vi "Day09-01_비전과 모션.vi"() -> ()   [LabVIEW 2021]
uses:
  <vilib>/userDefined/High Color/IMAQdx.ctl
  <vilib>/vision/driver/NI_Vision_Acquisition_Software.lvlib
  <vilib>/vision/NI_Vision_Development_Module.lvlib
panel:
  out "Image 3":T1(plugin-control)
  out "색상":enum16{"모름", "빨강", "초록", "노랑", "파랑", "보라", "하늘"}(ring)
  out "히스토그램":u8[][](graph)
  in  "수집 3":bool
  in  "정지 3":bool
  out "Image 2":T1(plugin-control)
  in  "정지 2":bool
  out "웨이브폼 그래프":u32[][](graph)
  in  "수집":bool
  in  "정지":bool
  out "Image":T1(plugin-control)
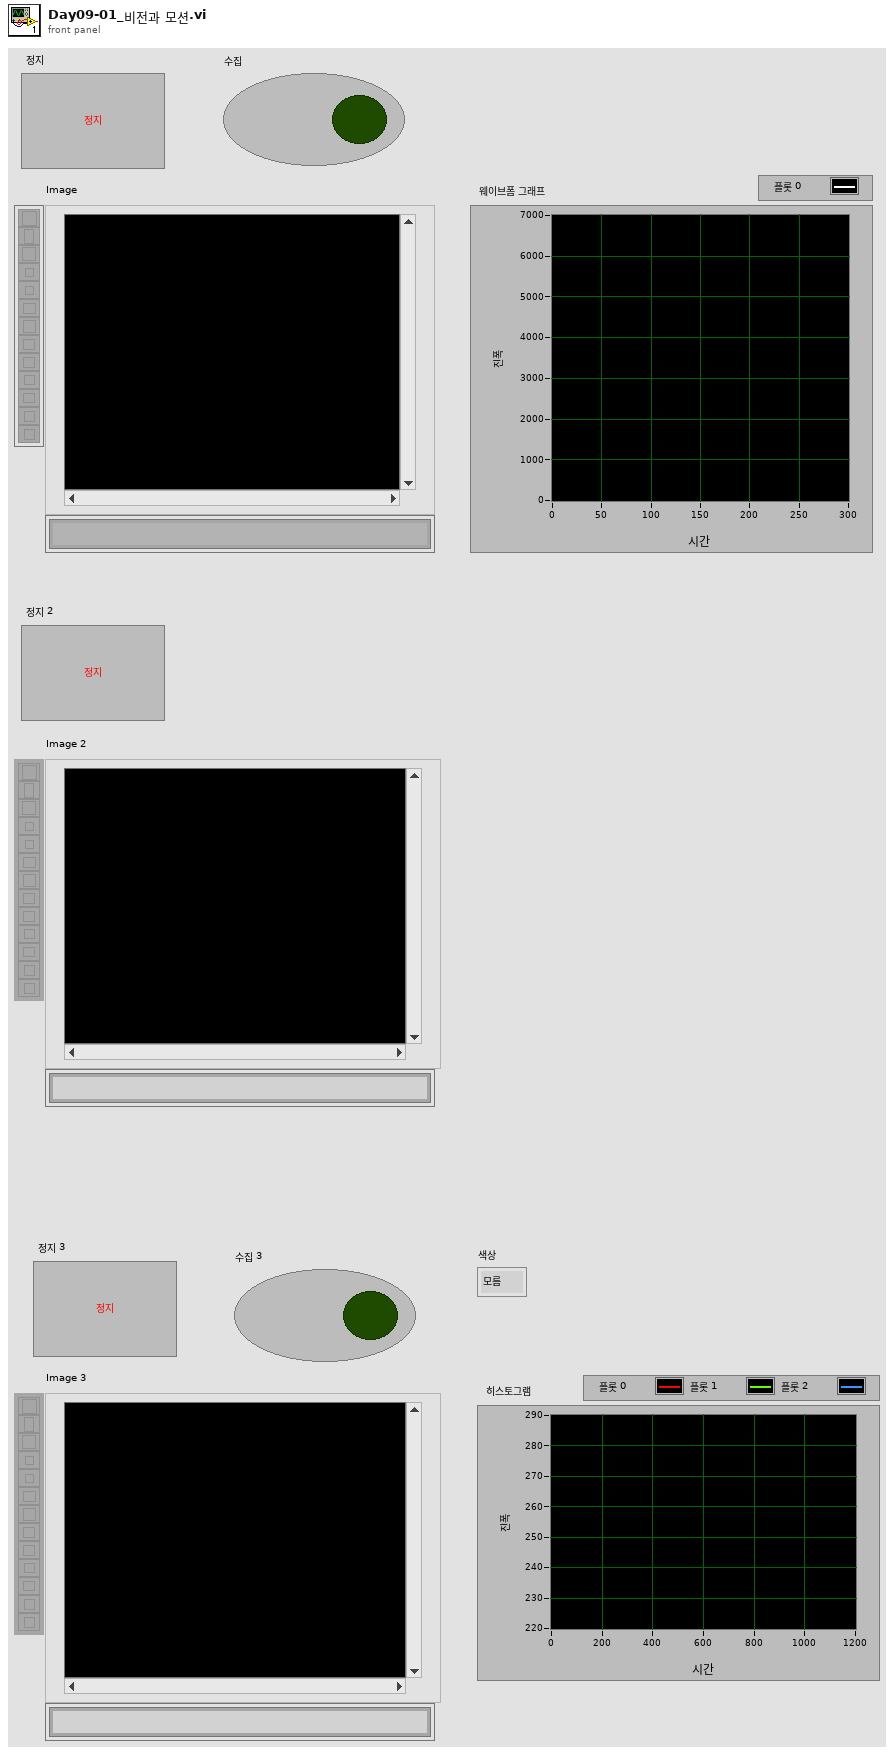
[diagram p1: front panel]
types:
  T1 = typedef "IMAQ Image.ctl" = refnum<image>
  T2 = typedef "IMAQdx.ctl" = refnum<k21>
  T3 = typedef "ROI Descriptor" = cluster{"Global Rectangle":i32[], "Contours":cluster{"ID":enum32{"External", "Internal"}, "Type":u32, "Coordinates":i32[]}[]}
  T4 = cluster{"histogram":u32[], "Minimal Value":sgl, "Maximal Value":sgl, "Starting Value":sgl, "Interval Width":sgl, "Mean Value":sgl, "Standard  Variation":sgl, "Area (pixels)":i32}
  T5 = enum16{"모름", "빨강", "초록", "노랑", "파랑", "보라", "하늘", "흰색"}[]
  T6 = enum16{"모름", "빨강", "초록", "노랑", "파랑", "보라", "하늘", "흰색"}
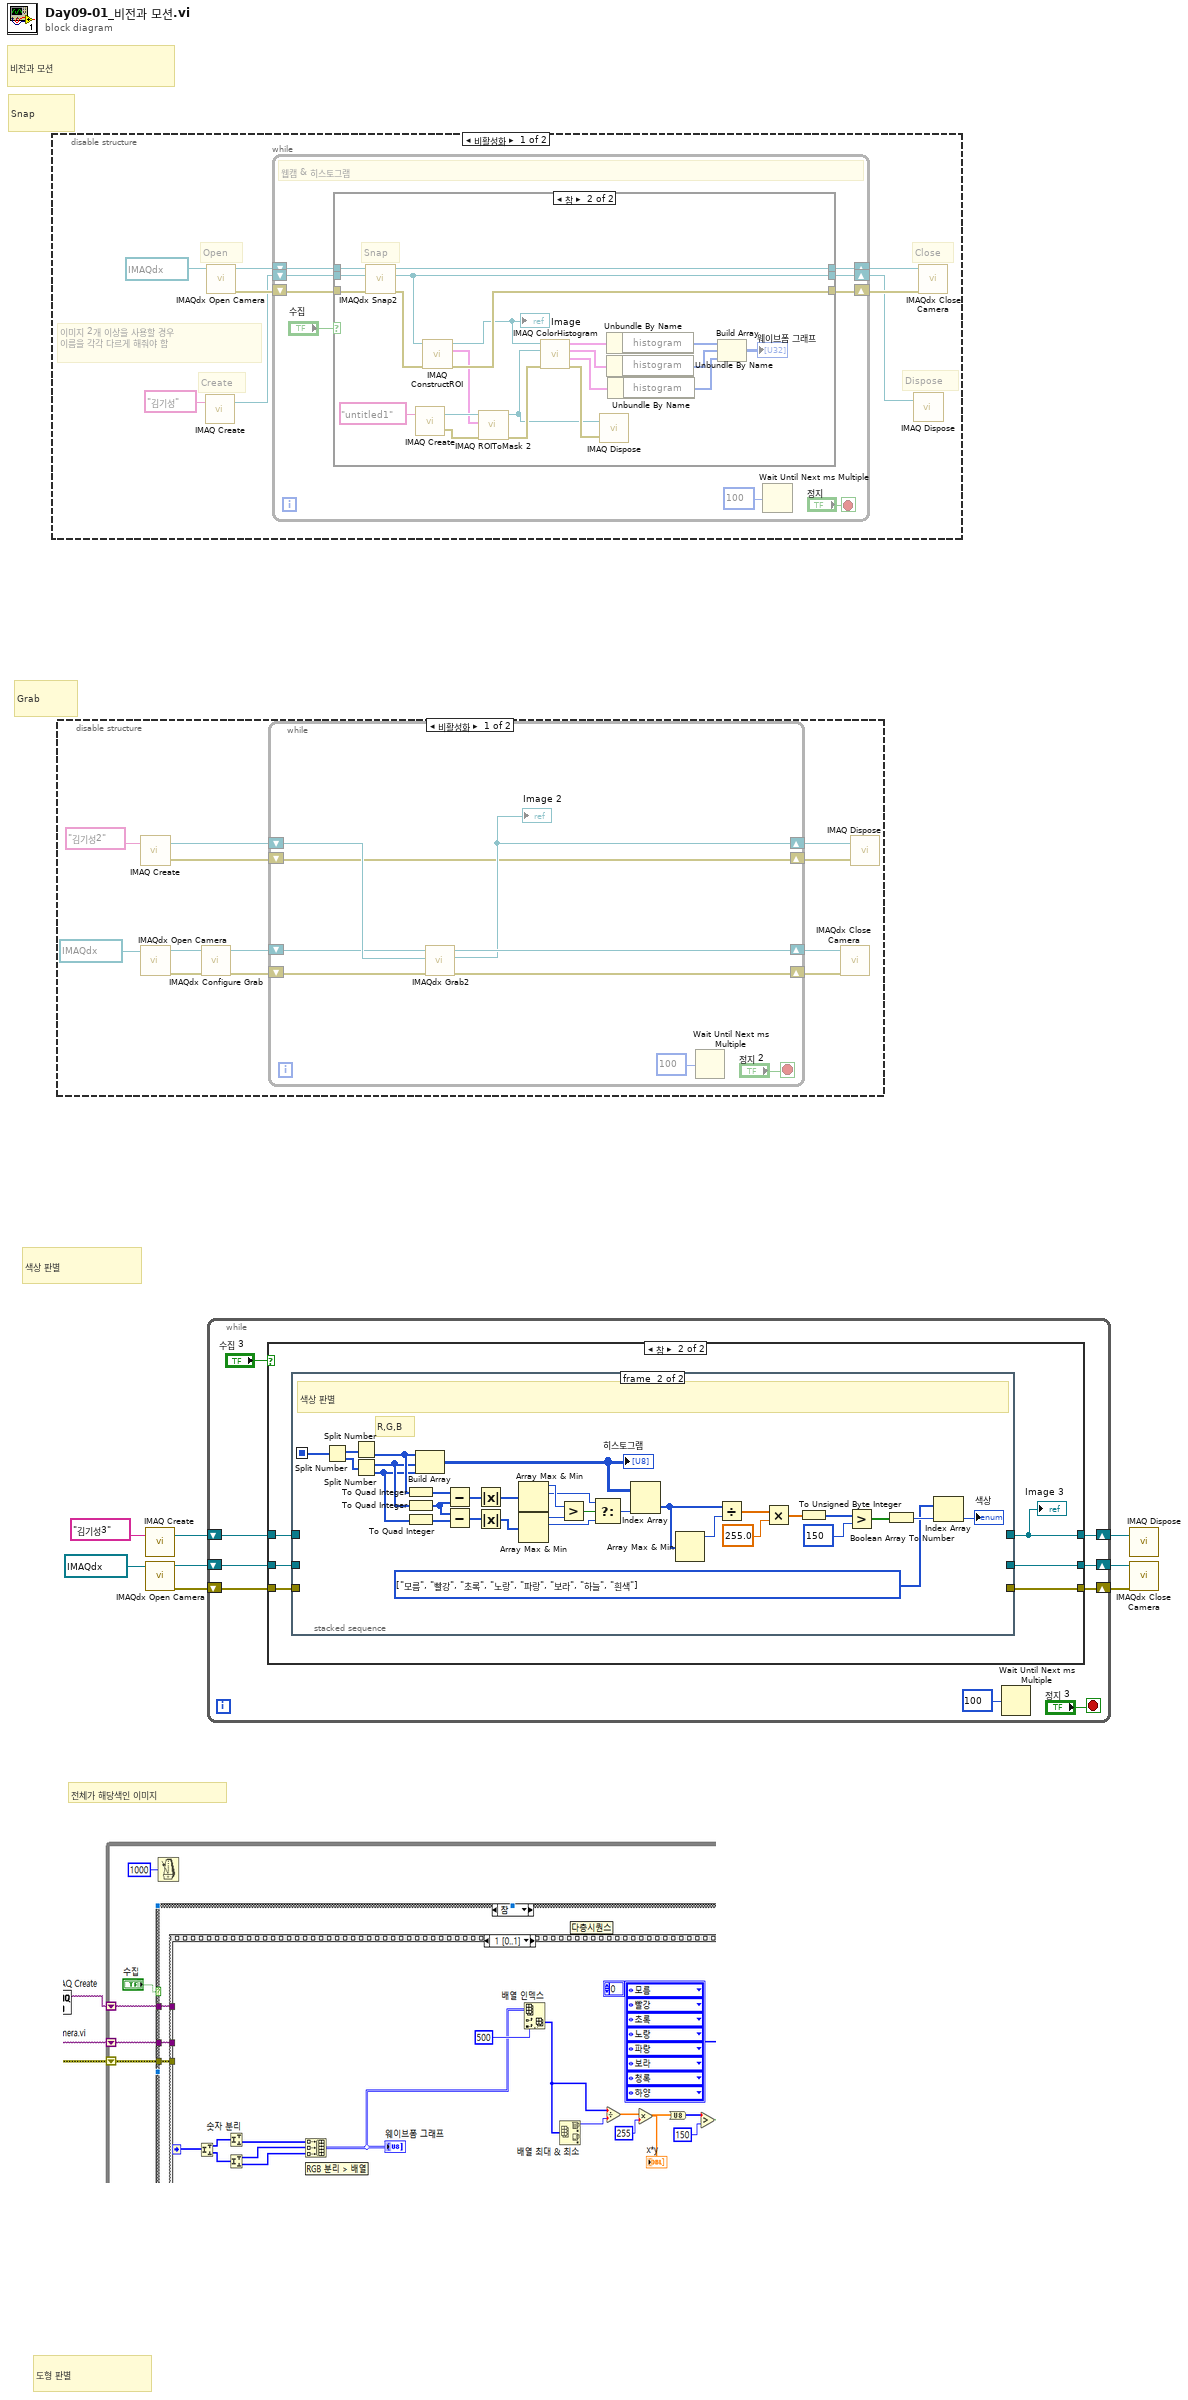
[diagram p0: block diagram]
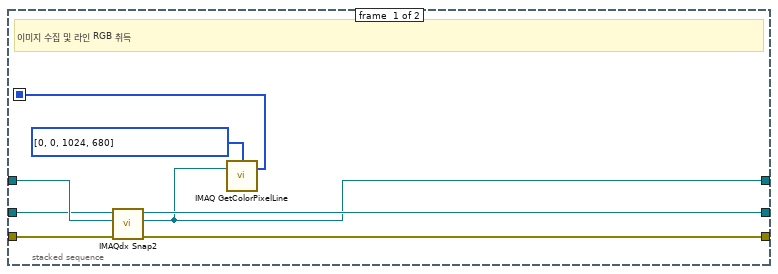
[diagram p4: hidden frame]
diagram:
  # "전체가 해당색인 이미지"
  # "도형 판별"
  # "색상 판별"
  # "Snap"
  # "Grab"
  # "비전과 모션"
  n1 = disable-structure shown="비활성화" {
    frame Disabled {
      # "Dispose"
      # "이미지 2개 이상을 사용할 경우\n이름을 각각 다르게 해줘야 함"
      # "Create"
      # "Close"
      # "Open"
      n2 = call "IMAQ Create"("Image Name"="김기성") -> ("New Image"=w10:T1)  [unwired: 4 in, 1 out]
      n3 = call <vilib>:"IMAQdx Open Camera.vi"("Session In"=T2 "cam1") -> ("error out"=w15:errorcluster, "Session Out"=w16:T2)  [unwired: 9 in]
      n4 = while {
        shift-right: [w23] -> w14
        shift-left: w16 -> [w25]
        shift-right: [w22] -> w13
        shift-left: w15 -> [w24]
        shift-right: [w18] -> w9
        shift-left: w10 -> [w21]
        stop <- "정지" stop-if-true
        # "웹캠 & 히스토그램"
        n5 = case shown="참" "수집" {
          tunnel: w25 -> [w28 w50]
          tunnel: w24 -> [w26 w49]
          tunnel: [w28 w48] -> w23
          tunnel: [w26 w39] -> w22
          tunnel: w21 -> [w27 w47]
          tunnel: [w27 w37] -> w18
          frame False {
          }
          frame True {
            # "Snap"
            n6 = call <vilib>:"IMAQdx Snap2.vi"("error in"=w49, "Image In"=w47, "Session In"=w50) -> ("error out"=w38:errorcluster, "Image Out"=w37:T1, "Session Out"=w48:T2)  [unwired: 6 in]
            n7 = call "IMAQ Create"("Image Name"="untitled1") -> ("New Image"=w35:T1, "error out"=w36:errorcluster)  [unwired: 4 in]
            n8 = call "IMAQ ConstructROI"("error in (no error)"=w38, "Image"=w37) -> ("error out"=w39:errorcluster, "ROI Descriptor Out"=w30:T3, "Image Out (duplicate)"=w29:T1)  [unwired: 6 in, 1 out]
            "Image" <- w29
            n9 = call "IMAQ ROIToMask 2"("error in (no error)"=w36, "ROI Descriptor"=w30, "Image"=w35) -> ("error out"=w33:errorcluster, "Image Out"=w31:T1)  [unwired: 6 in, 1 out]
            n10 = call "IMAQ ColorHistogram"("Image Src"=w29, "Image Mask"=w31, "error in (no error)"=w33) -> ("Red or Hue or X or L* Histogram Report"=w46:T4, "Green or Sat or Y or a* Histogram Report"=w45:T4, "Blue or Luma or Val or Inten or Z or b* Histogram Report"=w44:T4, "error out"=w32:errorcluster)  [unwired: 3 in]
            n11 = call "IMAQ Dispose"("Image"=w31, "error in (no error)"=w32) -> ()  [unwired: 4 in, 1 out]
            n12 = Unbundle By Name(w46) -> ("histogram"=w43:u32[])
            n13 = Unbundle By Name(w45) -> ("histogram"=w42:u32[])
            n14 = Unbundle By Name(w44) -> ("histogram"=w41:u32[])
            n15 = Build Array(w43, w42, w41) -> (→"웨이브폼 그래프":u32[][])
          }
        }
        n16 = Wait Until Next ms Multiple(millisecond multiple=u32 100 ("ms 배수")) -> ()  [unwired: 1 out]
      }
      n17 = call "IMAQ Dispose"("Image"=w9) -> ()  [unwired: 5 in, 1 out]
      n18 = call <vilib>:"IMAQdx Close Camera.vi"("error in"=w13, "Session In"=w14) -> ()  [unwired: 9 in, 1 out]
    }
    frame Enabled {
    }
  }
  n19 = disable-structure shown="비활성화" {
    frame Disabled {
      n20 = call "IMAQ Create"("Image Name"="김기성2") -> ("New Image"=w57:T1, "error out"=w51:errorcluster)  [unwired: 4 in]
      n21 = call <vilib>:"IMAQdx Open Camera.vi"("Session In"=T2 "cam1") -> ("error out"=w54:errorcluster, "Session Out"=w55:T2)  [unwired: 9 in]
      n22 = call <vilib>:"IMAQdx Configure Grab.vi"("error in"=w54, "Session In"=w55) -> ("error out"=w53:errorcluster, "Session Out"=w52:T2)  [unwired: 8 in]
      n23 = while {
        shift-right: [w63] -> w60
        shift-left: w51 -> [w63]
        shift-right: [w64] -> w59
        shift-left: w57 -> [w69]
        shift-right: [w70] -> w56
        shift-left: w52 -> [w68]
        shift-right: [w71] -> w58
        shift-left: w53 -> [w67]
        stop <- "정지 2" stop-if-true
        n24 = call <vilib>:"IMAQdx Grab2.vi"("error in"=w67, "Image In"=w69, "Session In"=w68) -> ("error out"=w71:errorcluster, "Image Out"=w64:T1, "Session Out"=w70:T2)  [unwired: 5 in, 1 out]
        "Image 2" <- w64
        n25 = Wait Until Next ms Multiple(millisecond multiple=u32 100 ("ms 배수")) -> ()  [unwired: 1 out]
      }
      n26 = call <vilib>:"IMAQdx Close Camera.vi"("error in"=w58, "Session In"=w56) -> ()  [unwired: 9 in, 1 out]
      n27 = call "IMAQ Dispose"("Image"=w59, "error in (no error)"=w60) -> ()  [unwired: 4 in, 1 out]
    }
    frame Enabled {
    }
  }
  n28 = call "IMAQ Create"("Image Name"="김기성3") -> ("New Image"=w7:T1)  [unwired: 4 in, 1 out]
  n29 = call <vilib>:"IMAQdx Open Camera.vi"("Session In"=T2 "cam2") -> ("error out"=w1:errorcluster, "Session Out"=w2:T2)  [unwired: 9 in]
  n30 = while {
    shift-right: [w72] -> w5
    shift-left: w7 -> [w78]
    shift-right: [w79] -> w8
    shift-left: w2 -> [w77]
    shift-right: [w80] -> w6
    shift-left: w1 -> [w76]
    stop <- "정지 3" stop-if-true
    n31 = case shown="참" "수집 3" {
      tunnel: [w81 w89] -> w80
      tunnel: [w82 w88] -> w79
      tunnel: w78 -> [w83 w87]
      tunnel: w77 -> [w82 w86]
      tunnel: w76 -> [w81 w85]
      tunnel: [w83 w84] -> w72
      frame False {
      }
      frame True {
        n32 = stacked-sequence {
          seq-local: [w90 _] -> [_ w128]
          tunnel: [w97 _] -> w89
          tunnel: [w96 _] -> w88
          tunnel: w87 -> [w95 _]
          tunnel: w86 -> [w94 _]
          tunnel: w85 -> [w93 _]
          tunnel: [w92 _] -> w84
          frame #0 {
            # "이미지 수집 및 라인 RGB 취득"
            n33 = call <vilib>:"IMAQdx Snap2.vi"("error in"=w93, "Image In"=w95, "Session In"=w94) -> ("error out"=w97:errorcluster, "Image Out"=w92:T1, "Session Out"=w96:T2)  [unwired: 6 in]
            n34 = call "IMAQ GetColorPixelLine"("Line Coordinates"=i32[] [0, 0, 1024, 680], "Image"=w92) -> ("Pixels Line (U32)"=w90:u32[])  [unwired: 2 in, 2 out]
          }
          frame #1 {
            w100 = T5 [enum."모름", enum."빨강", enum."초록", enum."노랑", enum."파랑", enum."보라", enum."하늘", enum."흰색"] items=["모름", "빨강", "초록", "노랑", "파랑", "보라", "하늘", "흰색"]
            # "R,G,B"
            # "색상 판별"
            n35 = Split Number(x=w128) -> (hi(x)=w127:u16[], lo(x)=w126:u16[])
            n36 = Split Number(x=w127) -> (lo(x)=w125:u8[])  [unwired: 1 out]
            n37 = Split Number(x=w126) -> (hi(x)=w124:u8[], lo(x)=w123:u8[])
            n38 = To Quad Integer(1:w125) -> (0:w122:i64[])
            n39 = To Quad Integer(1:w124) -> (0:w120:i64[])
            n40 = To Quad Integer(1:w123) -> (0:w121:i64[])
            n41 = Build Array(w125, w124, w123) -> (w110:u8[][])
            "히스토그램" <- w110
            n42 = Subtract(x=w122, y=w120) -> (x-y=w119:i64[])
            n43 = Subtract(x=w120, y=w121) -> (x-y=w118:i64[])
            n44 = Absolute Value(x=w119) -> (abs(x)=w117:i64[])
            n45 = Absolute Value(x=w118) -> (abs(x)=w116:i64[])
            n46 = Array Max & Min(array=w117) -> (max value=w114:i64, max index (indices)=w112:i32)  [unwired: 2 out]
            n47 = Array Max & Min(array=w116) -> (max value=w115:i64, max index (indices)=w111:i32)  [unwired: 2 out]
            n48 = Greater?(x=w114, y=w115) -> (0:w113:bool)
            n49 = Select(t=w112, s=w113, f=w111) -> (s? t:f=w99:i32)
            n50 = Index Array(array=w110, index (col)=w99) -> (element=w109:u8[])  [unwired: 1 in]
            n51 = Array Max & Min(array=w109) -> (max value=w108:u8)  [unwired: 3 out]
            n52 = Divide(x=w109, y=w108) -> (x/y=w107:dbl[])
            n53 = Multiply(x=w107, y=255.0) -> (x*y=w105:dbl[])
            n54 = To Unsigned Byte Integer(number=w105) -> (unsigned 8bit integer=w104:u8[])
            n55 = Greater?(x=w104, y=150) -> (0:w102:bool[])
            n56 = Boolean Array To Number(Boolean array=w102) -> (number=w101:u32)
            n57 = Index Array(array=w100, index=w101) -> (element=→"색상":T6)
          }
        }
        "Image 3" <- w84
      }
    }
    n58 = Wait Until Next ms Multiple(millisecond multiple=u32 100 ("ms 배수")) -> ()  [unwired: 1 out]
  }
  n59 = call "IMAQ Dispose"("Image"=w5) -> ()  [unwired: 5 in, 1 out]
  n60 = call <vilib>:"IMAQdx Close Camera.vi"("error in"=w6, "Session In"=w8) -> ()  [unwired: 9 in, 1 out]
